vi "Hood Manual Override.vi"(9 "Output":dbl, 10 "Hood Man. Request":bool, 11 "Hood Manual Value":dbl) -> (3 "Hood Output":dbl)   [LabVIEW 2015]
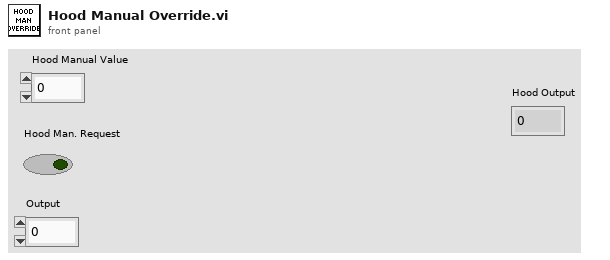
[diagram p1: front panel]
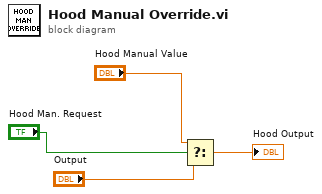
[diagram p0: block diagram]
diagram:
  n1 = Select(t="Hood Manual Value", s="Hood Man. Request", f="Output") -> (s? t:f=→"Hood Output":dbl)
